vi "test_windowsCamera.vi"() -> ()   [LabVIEW 2021]
uses:
  <vilib>/Analysis/Matrix/Datatypes/RealMatrix.ctl
  <vilib>/Analysis/Matrix/NI_Matrix.lvlib
panel:
  in  "stop":bool
  out "appended array":T1
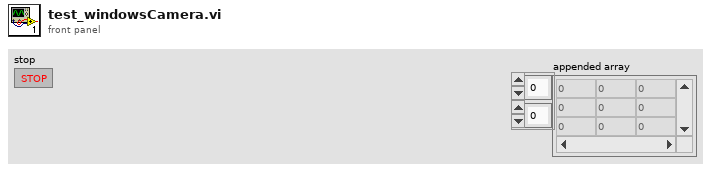
[diagram p1: front panel]
types:
  T1 = typedef "NI_Matrix.lvlib/RealMatrix.ctl" = dbl[][]
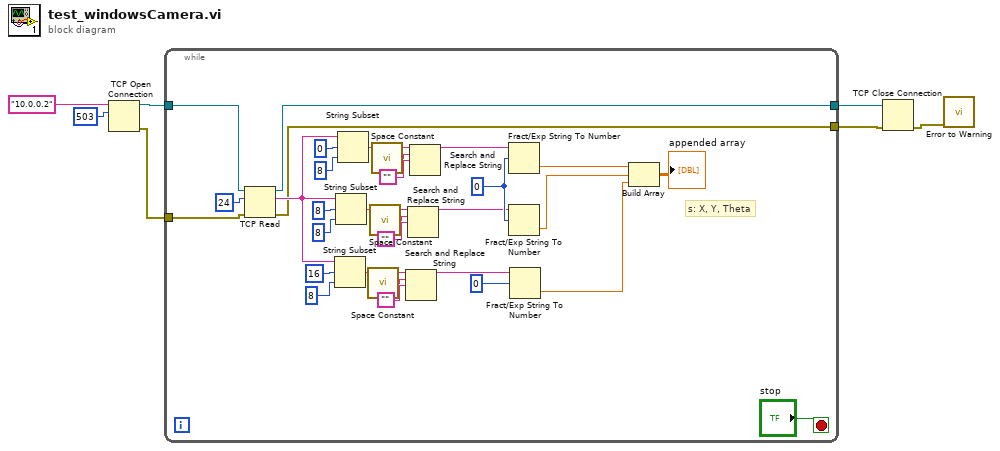
[diagram p0: block diagram]
diagram:
  n1 = TCP Open Connection(address="10.0.0.2", remote port or service name=u16 503) -> (connection ID=w5:refnum<k5>, error out=w3:errorcluster)  [unwired: 3 in]
  n2 = while {
    tunnel: w5 -> [w17]
    tunnel: [w13] -> w4
    tunnel: w3 -> [w10]
    tunnel: [w9] -> w2
    stop <- "stop" stop-if-true
    w38 = 0
    # "s: X, Y, Theta"
    n3 = TCP Read(connection ID=w17, bytes to read=24, error in (no error)=w10) -> (connection ID out=w13:refnum<k5>, data out=w19:string, error out=w9:errorcluster)  [unwired: 2 in]
    n4 = String Subset(string=w19, offset (0)=16, length (rest)=8 ("length (rest)")) -> (substring=w21:string)
    n5 = String Subset(string=w19, offset (0)=8, length (rest)=8 ("length (rest)")) -> (substring=w20:string)
    n6 = String Subset(string=w19, offset (0)=0, length (rest)=8 ("length (rest)")) -> (substring=w26:string)
    n7 = call <vilib>:"Space Constant.vi"() -> ("String"=w29:string)
    n8 = call <vilib>:"Space Constant.vi"() -> ("String"=w31:string)
    n9 = call <vilib>:"Space Constant.vi"() -> ("String"=w33:string)
    n10 = Search and Replace String(input string=w21, search string=w29, replace string="") -> (result string=w16:string)  [unwired: 5 in, 3 out]
    n11 = Search and Replace String(input string=w20, search string=w31, replace string="") -> (result string=w15:string)  [unwired: 5 in, 3 out]
    n12 = Search and Replace String(input string=w26, search string=w33, replace string="") -> (result string=w14:string)  [unwired: 5 in, 3 out]
    n13 = Fract/Exp String To Number(string=w14, offset=w38) -> (number=w37:dbl)  [unwired: 2 in, 1 out]
    n14 = Fract/Exp String To Number(string=w15, offset=w38) -> (number=w36:dbl)  [unwired: 2 in, 1 out]
    n15 = Fract/Exp String To Number(string=w16, offset=0) -> (number=w8:dbl)  [unwired: 2 in, 1 out]
    n16 = Build Array(w37, w36, w8) -> (→"appended array":T1)
  }
  n17 = TCP Close Connection(connection ID=w4, error in (no error)=w2) -> (error out=w1:errorcluster)  [unwired: 1 in, 1 out]
  n18 = call <vilib>:"Error to Warning.vi"("error in"=w1) -> ()  [unwired: 14 in, 1 out]
